vi "Obtain Broadcast Events.vi"(8 "error in (no error)":errorcluster, 10 "Create New?":bool) -> (0 "error out":errorcluster, 2 "Tool Module Broadcast Events":T1)   [LabVIEW 2015, in "Tool Module.lvlib"]
doc: "This VI Obtains/Creates the Broadcast events that will be used for other modules to register to receive messages from the module that owns this VI.\n\n<b>NOTE</b>: The contents of this VI are automatically generated and modified by the <b>Tools > Delacor > DQMH</b> utilities. Consider using those utilities instead of making your own modifications to this VI.\n_____\nBased on Delacor QMH Project Template 2.1.0.2."
uses:
  Tool Module.lvlib
  Broadcast Events--cluster.ctl
  Did Init Argument--cluster.ctl
  Status Updated Argument--cluster.ctl
  Error Reported Argument--cluster.ctl
  Stop Argument--cluster.ctl
  Get Module Execution Status Argument--cluster.ctl
  Send Status Argument--cluster.ctl
  Support/_STATUS Typedef--cluster.ctl
  Trigger Argument--cluster.ctl
  Connected Argument--cluster.ctl
  Read from File Rtn Argument--cluster.ctl
  Device Temperature Argument--cluster.ctl
  Tool Typedefs/_Temperature All Arrays--typedef.ctl
panel:
  # "NOTE: The contents of this VI are automatically generated and modified by the Tools > Delacor > DQMH utilities. Consider using those utilities instead of making your own modifications to this VI."
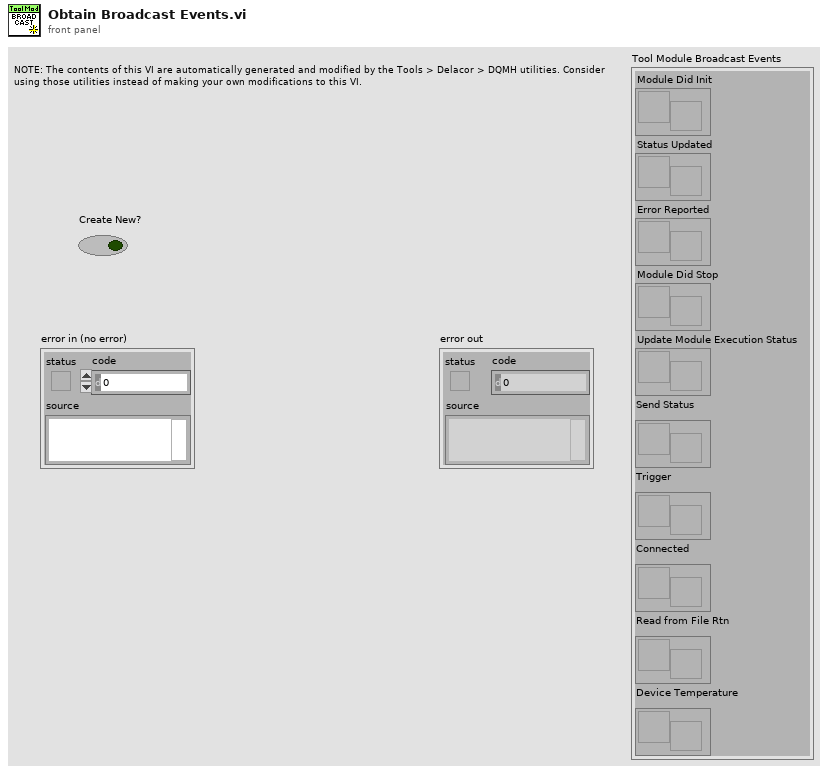
[diagram p1: front panel]
types:
  T1 = typedef "Tool Module.lvlib/Broadcast Events--cluster.ctl" = cluster{"Module Did Init":refnum<user-event>, "Status Updated":refnum<user-event>, "Error Reported":refnum<user-event>, "Module Did Stop":refnum<user-event>, "Update Module Execution Status":refnum<user-event>, "Send Status":refnum<user-event>, "Trigger":refnum<user-event>, "Connected":refnum<user-event>, "Read from File Rtn":refnum<user-event>, "Device Temperature":refnum<user-event>}
  T2 = typedef "Tool Module.lvlib/Device Temperature Argument--cluster.ctl" = cluster{"Device Temperature Arrays":T3}
  T3 = typedef "_Temperature All Arrays--typedef.ctl" = cluster{"Temp Sensors":dbl[], "High Thold ":dbl[], "Low Thold ":dbl[]}
  T4 = typedef "Tool Module.lvlib/Read from File Rtn Argument--cluster.ctl" = cluster{"Filename":string, "XML String":string, "Error Status":errorcluster}
  T5 = typedef "Tool Module.lvlib/Connected Argument--cluster.ctl" = cluster{"Connected":bool, "Tool Type":u16, "Tool SN":u16}
  T6 = typedef "Tool Module.lvlib/Trigger Argument--cluster.ctl" = cluster{"Trigger":bool}
  T7 = typedef "Tool Module.lvlib/Send Status Argument--cluster.ctl" = cluster{"STATUS":T8}
  T8 = typedef "Tool Module.lvlib/_STATUS Typedef--cluster.ctl" = cluster{"Initialized":bool, "Connected":bool, "Ready":bool, "Inspecting":bool, "Position":dbl, "Status":u16, "Error":bool, "Code":i32, "MC SM State":u16, "M_Ctrl":u16}
  T9 = typedef "Tool Module.lvlib/Get Module Execution Status Argument--cluster.ctl" = cluster{"Running?":bool}
  T10 = typedef "Tool Module.lvlib/Stop Argument--cluster.ctl" = cluster{"Origin":string, "Exit via Stop Module Req?":bool, "Wait for Module to stop?":bool}
  T11 = typedef "Tool Module.lvlib/Error Reported Argument--cluster.ctl" = cluster{"Error":errorcluster, "Additional Information":string, "Module Name":string}
  T12 = typedef "Tool Module.lvlib/Status Updated Argument--cluster.ctl" = cluster{"Status":string}
  T13 = typedef "Tool Module.lvlib/Did Init Argument--cluster.ctl" = cluster{"Init?":bool, "Info":string}
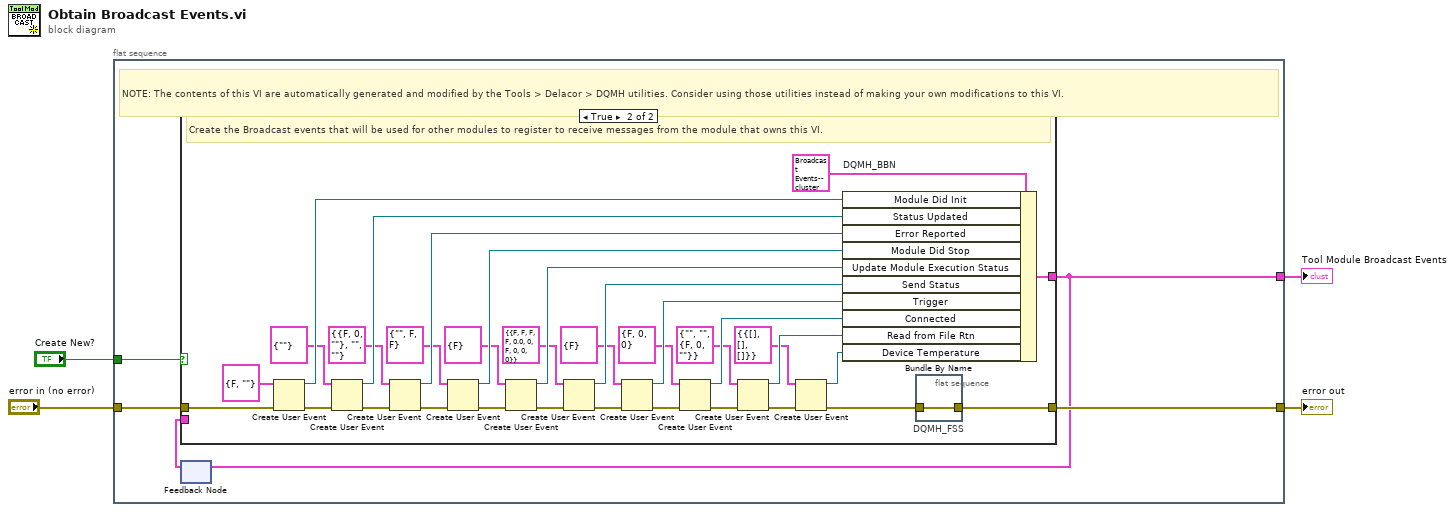
[diagram p0: block diagram]
diagram:
  n1 = flat-sequence {
    tunnel: [w9] -> w4
    tunnel: "error in (no error)" -> [w8]
    tunnel: [w6] -> w2
    tunnel: "Create New?" -> [w5]
    frame #0 {
      # "NOTE: The contents of this VI are automatically generated and modified by the Tools > Delacor > DQMH utilities. Consider using those utilities instead of making your own modifications to this VI."
      n2 = feedback #1() -> (w7:T1)  [unwired: 1 in]
      n3 = case shown="True" w5 {
        tunnel: [w10 w30] -> w9
        tunnel: w8 -> [w10 w45]
        tunnel: [w11 w42] -> w6
        tunnel: w7 -> [w11 _]
        frame False {
          # "Obtain the Broadcast events that were created in a previous call to this VI."
        }
        frame True {
          # "Create the Broadcast events that will be used for other modules to register to receive messages from the module that owns this VI."
          n4 = Create User Event(user event datatype=T13 {"Init?"=FALSE, "Info"=""} ("Did Init Argument"), error in=w45) -> (user event=w43:refnum<user-event>, error out=w40:errorcluster)
          n5 = Create User Event(user event datatype=T12 {"Status"=""} ("Status Updated Argument"), error in=w40) -> (user event=w37:refnum<user-event>, error out=w39:errorcluster)
          n6 = Create User Event(user event datatype=T11 {"Error"={"status"=FALSE, "code"=0, "source"=""}, "Additional Information"="", "Module Name"=""} ("Error Reported Argument"), error in=w39) -> (user event=w34:refnum<user-event>, error out=w36:errorcluster)
          n7 = Create User Event(user event datatype=T10 {"Origin"="", "Exit via Stop Module Req?"=FALSE, "Wait for Module to stop?"=FALSE} ("Stop Argument"), error in=w36) -> (user event=w32:refnum<user-event>, error out=w31:errorcluster)
          n8 = Create User Event(user event datatype=T9 {"Running?"=FALSE} ("Get Module Execution Status Argument"), error in=w31) -> (user event=w28:refnum<user-event>, error out=w29:errorcluster)
          n9 = Create User Event(user event datatype=T7 {"STATUS"={"Initialized"=FALSE, "Connected"=FALSE, "Ready"=FALSE, "Inspecting"=FALSE, "Position"=0.0, "Status"=0, "Error"=FALSE, "Code"=0, "MC SM State"=0, "M_Ctrl"=0}} ("Send Status Argument"), error in=w29) -> (user event=w25:refnum<user-event>, error out=w26:errorcluster)
          n10 = Create User Event(user event datatype=T6 {"Trigger"=FALSE} ("Trigger Argument"), error in=w26) -> (user event=w22:refnum<user-event>, error out=w23:errorcluster)
          n11 = Create User Event(user event datatype=T5 {"Connected"=FALSE, "Tool Type"=0, "Tool SN"=0} ("Connected Argument"), error in=w23) -> (user event=w20:refnum<user-event>, error out=w18:errorcluster)
          n12 = Create User Event(user event datatype=T4 {"Filename"="", "XML String"="", "Error Status"={"status"=FALSE, "code"=0, "source"=""}} ("Read from File Rtn Argument"), error in=w18) -> (user event=w16:refnum<user-event>, error out=w17:errorcluster)
          n13 = Create User Event(user event datatype=T2 {"Device Temperature Arrays"={"Temp Sensors"=[], "High Thold "=[], "Low Thold "=[]}} ("Device Temperature Argument"), error in=w17) -> (user event=w13:refnum<user-event>, error out=w14:errorcluster)
          n14 = Bundle By Name "DQMH_BBN"(cluster=T1 {"Module Did Init"=refnum, "Status Updated"=refnum, "Error Reported"=refnum, "Module Did Stop"=refnum, "Update Module Execution Status"=refnum, "Send Status"=refnum, "Trigger"=refnum, "Connected"=refnum, "Read from File Rtn"=refnum, "Device Temperature"=refnum} ("output cluster"), "Module Did Init"=w43, "Status Updated"=w37, "Error Reported"=w34, "Module Did Stop"=w32, "Update Module Execution Status"=w28, "Send Status"=w25, "Trigger"=w22, "Connected"=w20, "Read from File Rtn"=w16, "Device Temperature"=w13) -> (w42:T1)
          n15 = flat-sequence "DQMH_FSS" {
            tunnel: w14 -> [w46]
            tunnel: [w46] -> w30
            frame #0 {
            }
          }
        }
      }
      n16 = feedback-in #1(w6) -> ()
    }
  }
  "Tool Module Broadcast Events" <- w2
  "error out" <- w4
